vi "Tosca-Demo Pretrial.vi"(0 "Args":string[](array[string]), 11 "error in (no error)":errorcluster) -> (15 "error out":errorcluster)   [LabVIEW 2015]
panel:
  out "data":T1
  in  "config":T1
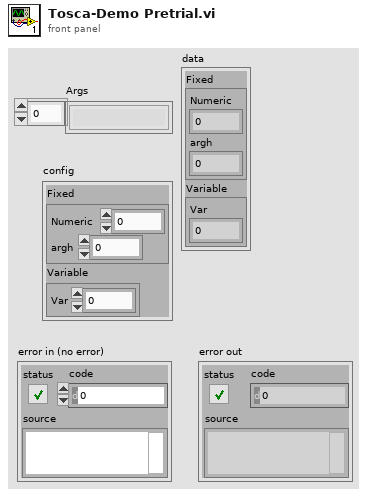
[diagram p1: front panel]
types:
  T1 = cluster{"Fixed":cluster{"Numeric":dbl, "argh":dbl}, "Variable":cluster{"Var":dbl}}
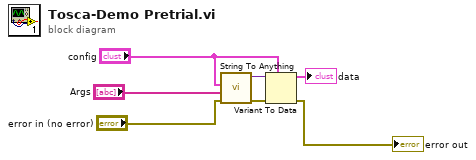
[diagram p0: block diagram]
diagram:
  n1 = call "String To Anything.vi"("Error In"="error in (no error)", "Strings"="Args", "Type of Anything"="config") -> ("Error Out"=w5:errorcluster, "Variant"=w4:variant)  [unwired: 7 in]
  n2 = Variant To Data(error in=w5, type="config", Variant=w4) -> (data=→"data":T1, error out=→"error out":errorcluster)
